vi "LM model function and gradient (2-Exp, Convolved, Periodic) v3.vi"(3 "output control":T1, 4 "data":variant, 5 "X":dbl[](array[numeric]), 6 "a":dbl[](array[numeric])) -> (0 "error out":errorcluster, 1 "f'(X,a)":dbl[][](array[numeric]), 2 "f(X,a)":dbl[](array[numeric]))   [LabVIEW 2021, in "Fits.lvlib"]
doc: "This template is the starting point for creating a model function to be passed to the Nonlinear Curve Fit.vi."
uses:
  Fits.lvlib
  <vilib>/gmath/NumericalOptimization/LM_output select.ctl
  Fit Control Data.ctl
  Graphs/XY Graph/XY Graph Plot Data.ctl
  1-Exp Parameters.ctl
  e69e6f48-ad21-4fab-bc0f-ff4b1b8ea852.vi
  Graphs/XY Graph/XY Graph Add-Ons.lvlib
  <vilib>/gmath/NI_Gmath.lvlib
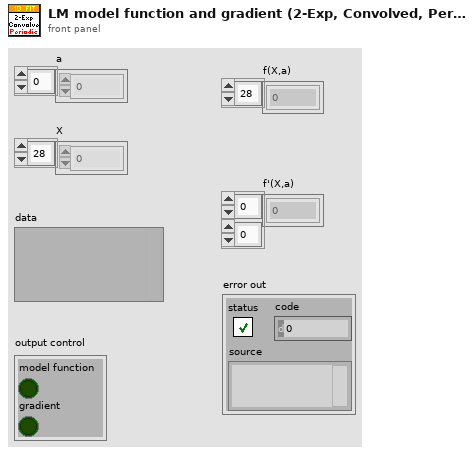
[diagram p1: front panel]
types:
  T1 = typedef "NI_Gmath.lvlib/LM_output select.ctl" = cluster{"model function":bool, "gradient":bool}
  T2 = typedef "Fits.lvlib/1-Exp Parameters.ctl" = cluster{"t_0":dbl, "B":dbl, "A":dbl, "tau":dbl, "T":dbl, "sigma":dbl}
  T3 = typedef "Fits.lvlib/Fit Control Data.ctl" = cluster{"IRF":T4, "Laser Period":dbl, "SYNC Period":dbl}
  T4 = typedef "XY Graph Add-Ons.lvlib/XY Graph Plot Data.ctl" = cluster{"X Array":dbl[], "Y Array":dbl[]}
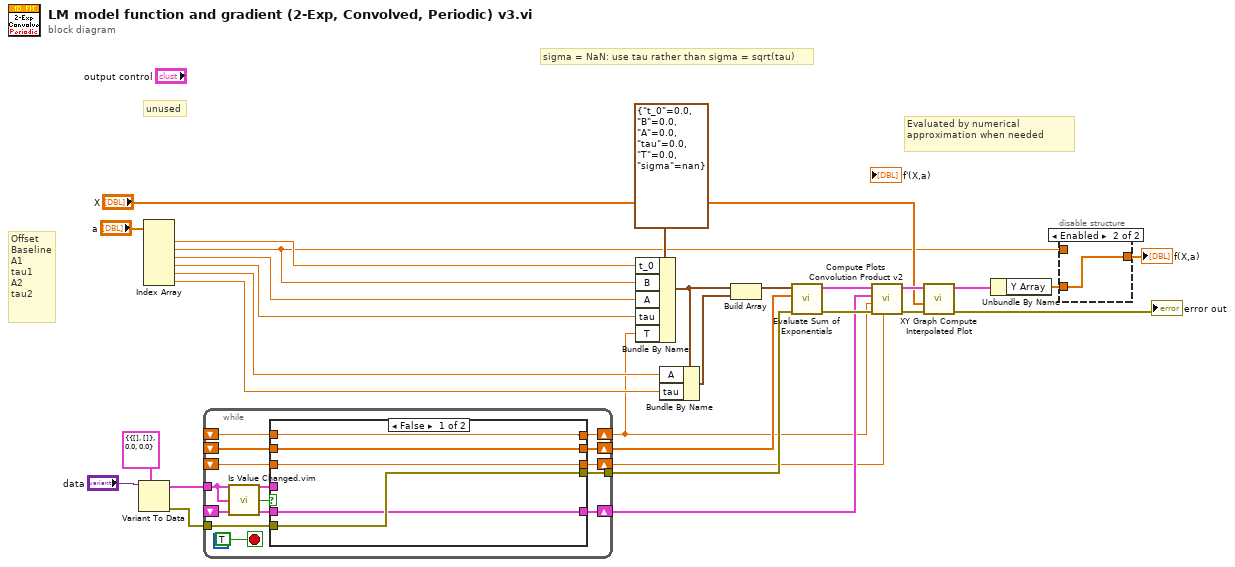
[diagram p0: block diagram]
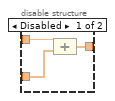
[diagram p2: hidden frame]
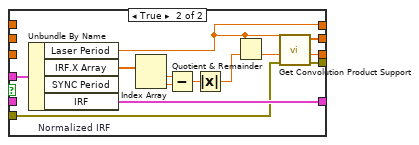
[diagram p3: hidden frame]
diagram:
  # "sigma = NaN: use tau rather than sigma = sqrt(tau)"
  # "unused"
  # "Evaluated by numerical approximation when needed"
  # "Offset\nBaseline\nA1\ntau1\nA2\ntau2"
  n1 = Variant To Data(type=T3 {"IRF"={"X Array"=[], "Y Array"=[]}, "Laser Period"=0.0, "SYNC Period"=0.0} ("Fit Control Data"), Variant="data") -> (data=w17:T3, error out=w16:errorcluster)  [unwired: 1 in]
  n2 = Index Array(array="a") -> (element #1=w26:dbl, element #2=w3:dbl, element #3=w24:dbl, element #4=w23:dbl, element #5=w21:dbl, element #6=w20:dbl)  [unwired: 6 in]
  n3 = while {
    tunnel: w17 -> [w38]
    tunnel: w16 -> [w41]
    tunnel: [w40] -> w9
    shift-right: [w39] -> w10
    shift-left: _ -> [w36]
    shift-right: [w42] -> w4
    shift-left: _ -> [w35]
    shift-right: [w34] -> w2
    shift-left: _ -> [w33]
    shift-right: [w31] -> w1
    shift-left: _ -> [w30]
    stop <- TRUE stop-if-true
    n4 = call "Is Value Changed.vim"("value"=w38) -> ("changed or first call?"=w32:bool)
    n5 = case shown="False" w32 {
      tunnel: [w45 w60] -> w42
      tunnel: w41 -> [w46 w54]
      tunnel: [w46 w53] -> w40
      tunnel: [w47 w52] -> w39
      tunnel: w38 -> [_ w51]
      tunnel: w36 -> [w47 _]
      tunnel: w35 -> [w45 _]
      tunnel: [w44 w50] -> w34
      tunnel: w33 -> [w44 _]
      tunnel: [w43 w48] -> w31
      tunnel: w30 -> [w43 _]
      frame False {
      }
      frame True {
        n6 = Unbundle By Name "Normalized IRF"(w51) -> ("Laser Period"=w50:dbl, "IRF.X Array"=w59:dbl[], "IRF"=w60:T4)  [unwired: 1 out]
        n7 = Index Array(array=w59) -> (element #1=w58:dbl, element #2=w57:dbl)  [unwired: 2 in]
        n8 = Subtract(x=w58, y=w57) -> (x-y=w56:dbl)
        n9 = Absolute Value(x=w56) -> (abs(x)=w49:dbl)
        n10 = Quotient & Remainder(x=w50, y=w49) -> (floor(x/y)=w55:dbl)  [unwired: 1 out]
        n11 = call "Get Convolution Product Support.vi"("Error In"=w54, "# Values"=w55, "IRF Period"=w50) -> ("Error Out"=w53:errorcluster, "Step"=w48:dbl, "Ramp"=w52:dbl[])  [unwired: 6 in]
      }
    }
  }
  n12 = Bundle By Name(cluster=T2 {"t_0"=0.0, "B"=0.0, "A"=0.0, "tau"=0.0, "T"=0.0, "sigma"=nan} ("1-Exp Parameters"), "t_0"=w26, "B"=w3, "A"=w24, "tau"=w23, "T"=w2) -> (w18:T2)
  n13 = Bundle By Name(cluster=w18, "A"=w21, "tau"=w20) -> (w19:T2)
  n14 = Build Array(w18, w19) -> (w11:T2[])
  n15 = call "Evaluate Sum of Exponentials.vi"("error in (no error)"=w9, "Ramp"=w10, "Exp Parameters Array"=w11) -> ("error out"=w12:errorcluster, "Plot"=w5:T4)  [unwired: 7 in]
  n16 = call "Compute Plots Convolution Product v2.vi"("Step"=w1, "Error In"=w12, "Period"=w2, "Plot 2 (kernel)"=w4, "Plot 1 (function)"=w5) -> ("Error Out"=w15:errorcluster, "Convolution Product"=w13:T4)  [unwired: 4 in, 1 out]
  n17 = call "XY Graph Compute Interpolated Plot.vi"("Error In"=w15, "Ramp"="X", "Plot"=w13) -> ("Error Out"=→"error out":errorcluster, "Interpolated Plot"=w14:T4)  [unwired: 7 in]
  n18 = Unbundle By Name(w14) -> ("Y Array"=w8:dbl[])
  n19 = disable-structure shown="Enabled" {
    disable-tunnel: [w63 w64] -> w25
    disable-tunnel: w8 -> [w62 w64]
    disable-tunnel: w3 -> [w61 _]
    frame Disabled {
      n20 = Compound Arithmetic op=ADD(w61, w62) -> (w63:dbl[])
    }
    frame Enabled {
    }
  }
  "f(X,a)" <- w25
